vi "myRIOXC Read Pin Name.vi"(7 "Size":i32, 8 "error in":errorcluster, 9 "Path":path, 11 "Connector":string) -> (0 "error out":errorcluster, 3 "Default Names":string[](array[string]))   [LabVIEW 2021]
doc: "This VI reads Pin name from \"Config.ini\" based on Connector Type,\nPin Peripheral and Pin Number."
uses:
  <vilib>/Utility/config.llb/Read Key (String).vi
  <vilib>/Utility/config.llb/NI_LVConfig.lvlib
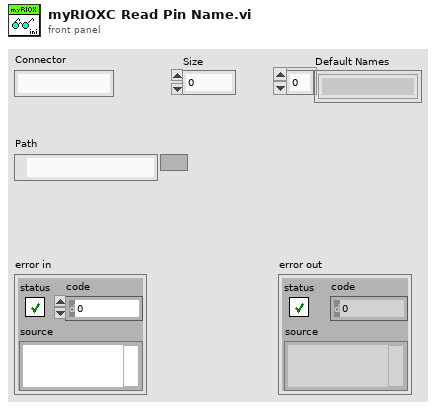
[diagram p1: front panel]
types:
  T1 = typedef "NI_LVConfig.lvlib/Config Data RefNum.ctl" = refnum<k1>
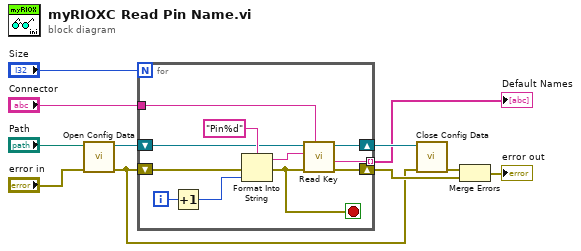
[diagram p0: block diagram]
diagram:
  n1 = call <vilib>:"Open Config Data.vi"("error in (no error)"="error in", "configuration file path"="Path") -> ("error out"=w2:errorcluster, "refnum"=w10:T1)  [unwired: 7 in, 1 out]
  n2 = for {
    N: "Size" -> [_]
    shift-right: [w18] -> w3
    shift-left: w2 -> [w17]
    shift-right: [w19] -> w11
    shift-left: w10 -> [w20]
    tunnel: [w16] -> w6 mode=indexing
    tunnel: "Connector" -> [w15]
    i -> [w14]
    stop <- w12 stop-if-true
    n3 = Increment(x=w14) -> (x+1=w13:i32)
    n4 = Format Into String(format string="Pin%d", error in=w17, w13) -> (resulting string=w22:string, error out=w12:errorcluster)  [unwired: 1 in]
    n5 = call-poly <vilib>:"Read Key.vi"("section"=w15, "error in (no error)"=w12, "key"=w22, "refnum"=w20) -> ("error out"=w18:errorcluster, "value"=w16:string, "refnum out"=w19:T1)  [unwired: 4 in, 1 out]
  }
  "Default Names" <- w6
  n6 = call <vilib>:"Close Config Data.vi"("error in (no error)"=w2, "refnum"=w11) -> ("error out"=w4:errorcluster)  [unwired: 8 in, 1 out]
  n7 = Merge Errors(w4, w3) -> (→"error out":errorcluster)
